vi "1-DSpecViewAndFit.vi"() -> ()   [LabVIEW 2022 SP3]
uses:
  <vilib>/Utility/file.llb/Read From Spreadsheet File (DBL).vi
  <vilib>/Utility/file.llb/Write To Spreadsheet File (DBL).vi
panel:
  in  "Extra File Att":dbl format="%.2f"
  out "single case fit data":T1 {"pts in fit" format="%.2f"; "midband fit" format="%.2f"; "intercept (b)" format="%.2f"; "slope (m)" format="%.3f"}
  in  "Log scaling?":bool=TRUE
  out "raw x coord":dbl[][](array[numeric]) format="%.2f"
  out "raw y coord":dbl[][](array[numeric]) format="%.2f"
  out "raw sector image":dbl[][](array[numeric]) format="%.2f"
  out "Axis scaling Params":T2 {"Y high" format="%.2f"; "Y low" format="%.2f"; "X left" format="%.2f"; "X right" format="%.2f"}
  out "Sector as data array":dbl[][](graph)
  in  "Last sector file":path
  in  "View Header?":bool
  in  "Save to Spectra.txt?":bool
  out "Cal File Att":string
  out "RF File Att":string
  in  "FFT size for":u16(ring)=6 items=["next 2^n", "8", "16", "32", "64", "128", "256", "512", "1024"]
  in  "Cal File Selection":u16(ring) items=["Don't subtract a Cal File", "Use Info in Header", "Specify Cal Info", "Make New Cal File"]
  in  "Cal File Name":string
  in  "Save New Cal File?":bool
  out "actual length\nof padded ROI":i32
  out "need this# of RF pts\nmatch Cal File":i32
  in  "Fit band":T3={"start"=3.5, "stop freq"=8.0, "center freq"=5.75} {"center freq" format="%.2f"; "stop freq" format="%.2f"; "start" format="%.2f"}
  out "Spectrum (dBr vs. MHz)":T4(graph)
  out "Raw data":i16[][](graph)
  in  "new eye file path":path
  # "Select region for spectrum analysis.\nKeep RED curser above and to left of blue.\nBath cursors can be on the same line."
  # "© 2000 Riverside Research Institute"
  # "Spectrum Fit Parameters"
  # "Blue curser controls upper right of sector ROI,\nRed curser controls lower left."
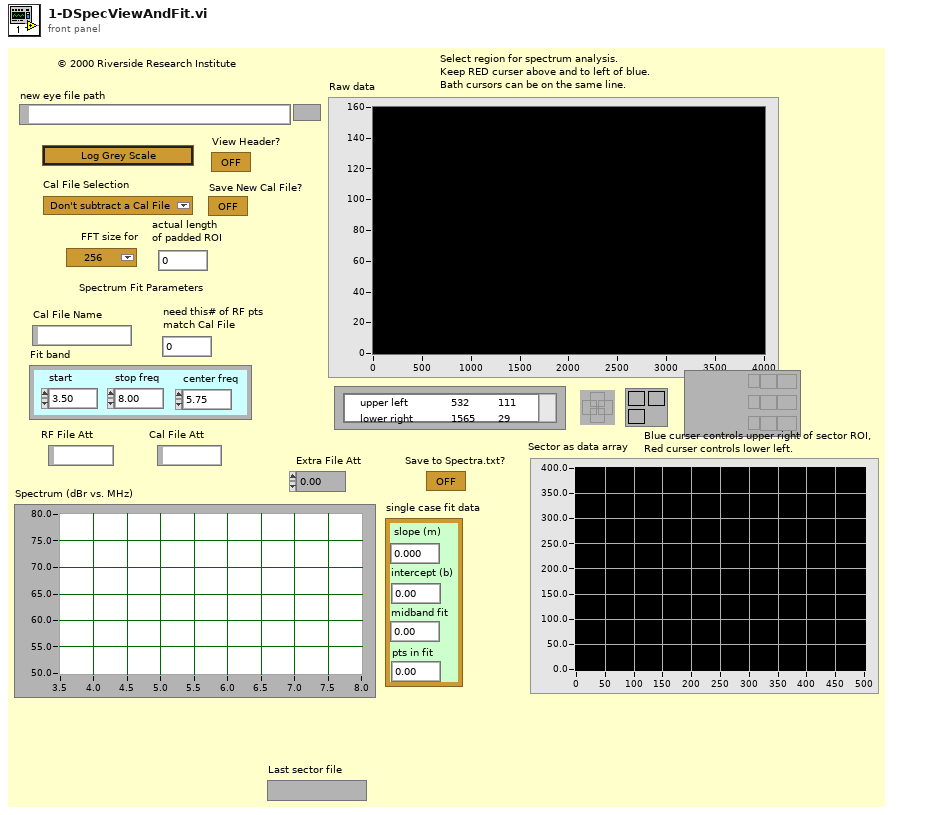
[diagram p1: front panel]
types:
  T1 = cluster{"slope (m)":dbl, "intercept (b)":dbl, "midband fit":dbl, "pts in fit":dbl}
  T2 = cluster{"X right":dbl, "X left":dbl, "Y low":dbl, "Y high":dbl}
  T3 = cluster{"start":dbl, "stop freq":dbl, "center freq":dbl}
  T4 = cluster{"fo of fit":dbl, "df (MHz)":dbl, "Best Linear Fit":dbl[]}[]
  T5 = cluster{"# rf points per line":u16, "# lines per scan":u16, "sample rate MHz":u16, "# A/D bits":u16, "# bytes per A/D":u16, "TGC Flag":u16, "A/D Type":string}
  T6 = cluster{"bandwidth":sgl, "center freq":sgl, "start freq":sgl, "ID":i32}
  T7 = cluster{"delay":sgl, "pivot distance":sgl, "sector scan angle":sgl, "operator":string, "Scan Mode":string, "location":string}
  T8 = cluster{"RF file name":string, "RF file att":string, "RF cal file name":string, "RF cal file att":string}
  T9 = cluster{"Cursor.Cursor X":dbl, dbl, "Cursor.Cursor Y":dbl, dbl}
  T10 = cluster{"Cursor.Cursor X":i32, i32, "Cursor.Cursor Y":i32, i32}
  T11 = cluster{"RF file name":string, "RF file att":string, "Cal File Name":string, "RF cal file att":string}
  T12 = cluster{"start freq":sgl, sgl, "center freq":sgl}
  T13 = cluster{"slope (m)":dbl[][], "intercept (b)":dbl[][], "midband fit":dbl[][], "pts in fit":dbl}
  T14 = cluster{"fo of fit":dbl, "df (MHz)":dbl, dbl[]}[]
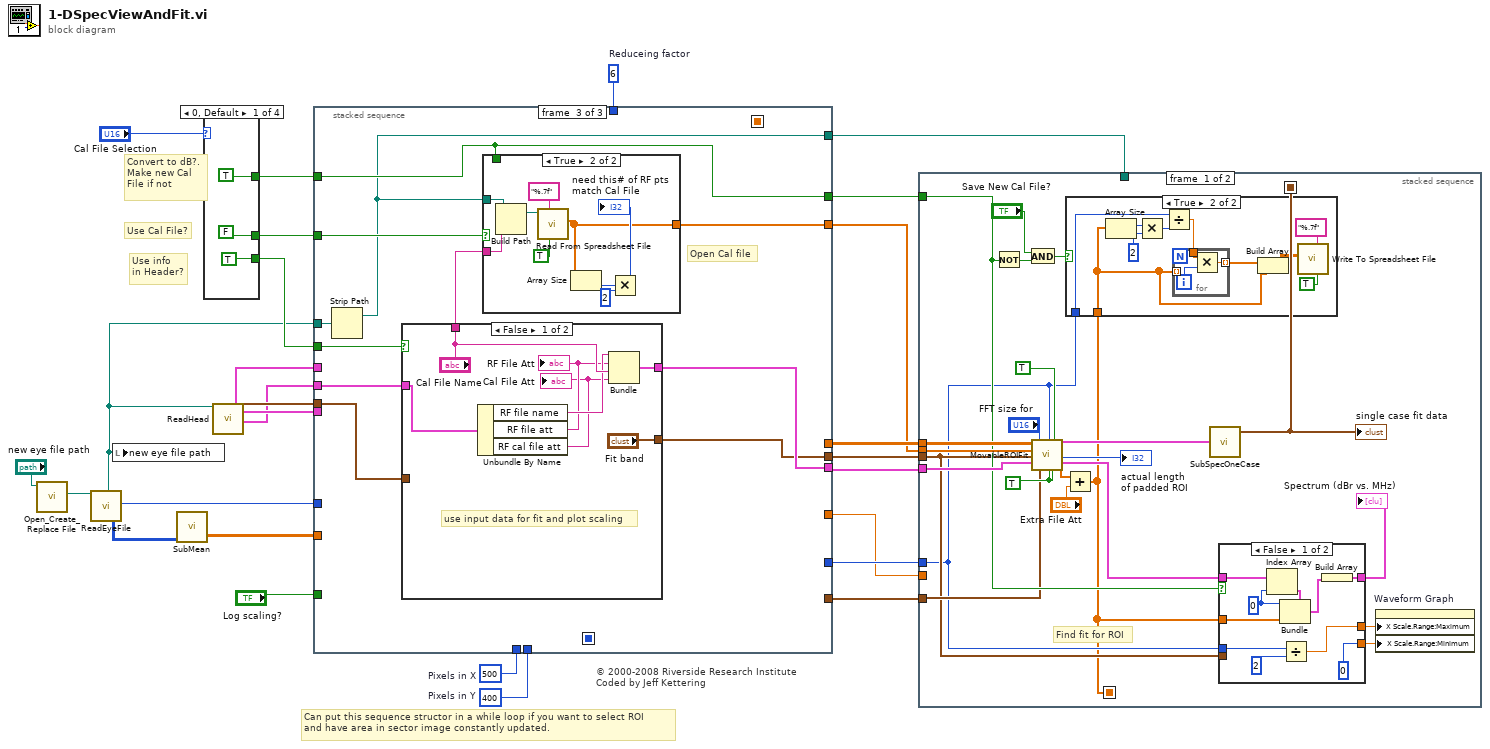
[diagram p0: block diagram]
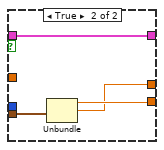
[diagram p2: hidden frame]
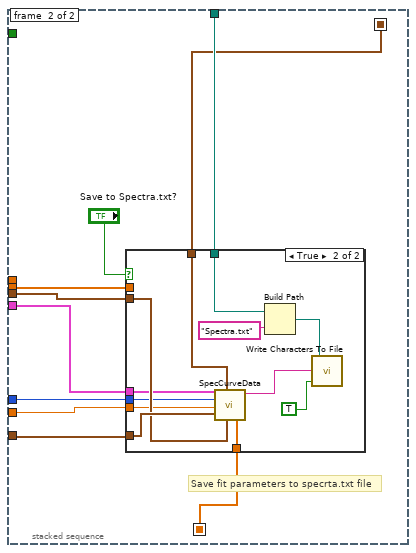
[diagram p4: hidden frame]
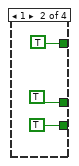
[diagram p6: hidden frame]
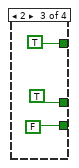
[diagram p7: hidden frame]
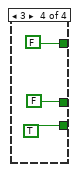
[diagram p8: hidden frame]
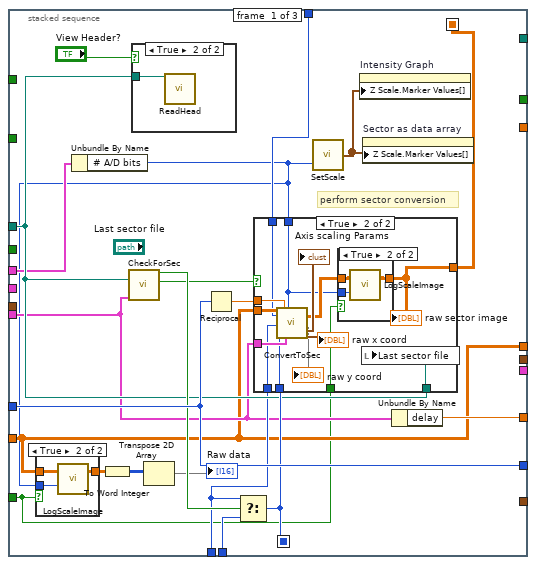
[diagram p9: hidden frame]
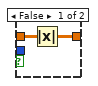
[diagram p10: hidden frame]
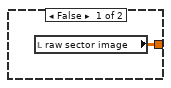
[diagram p12: hidden frame]
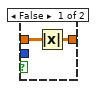
[diagram p13: hidden frame]
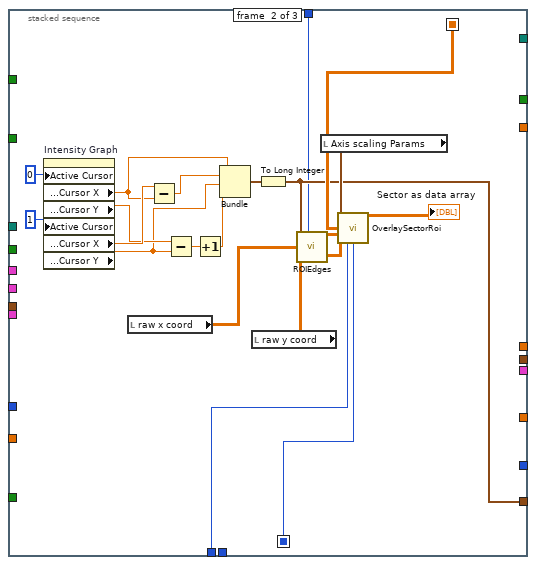
[diagram p14: hidden frame]
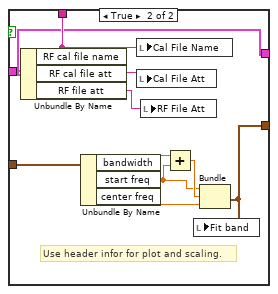
[diagram p15: hidden frame]
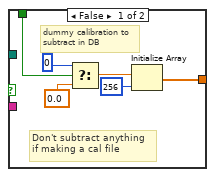
[diagram p16: hidden frame]
diagram:
  w7 = 400  # Pixels in Y
  w6 = 500  # Pixels in X
  w8 = 6  # Reduceing factor
  # "© 2000-2008 Riverside Research Institute\nCoded by Jeff Kettering"
  # "Can put this sequence structor in a while loop if you want to select ROI\nand have area in sector image constantly updated."
  # "Convert to dB?.\nMake new Cal\nFile if not"
  # "Use Cal File?"
  # "Use info\nin Header?"
  n1 = call <vilib>:"Open_Create_Replace File.vi"("file path"="new eye file path") -> ("new file path"=w13:path)  [unwired: 5 in, 5 out]
  n2 = call "ReadEyeFile.vi"("new file path"=w13) -> ("new path out"=w2:path, "2-D data array"=w3:i16[][], "sample rate MHz"=w23:u16)  [unwired: 1 in, 15 out]
  n3 = local write "new eye file path"(w2) -> ()
  n4 = call "SubMean.vi"("Scan Data In"=w3) -> ("Array"=w1:dbl[][])  [unwired: 3 in, 1 out]
  n5 = case shown="0, Default" "Cal File Selection" {
    tunnel: [TRUE TRUE TRUE FALSE] -> w26
    tunnel: [FALSE TRUE TRUE FALSE] -> w4
    tunnel: [TRUE TRUE FALSE TRUE] -> w25
    frame 0, Default {
    }
    frame 1 {
    }
    frame 2 {
    }
    frame 3 {
    }
  }
  n6 = call "ReadHead.vi"("new file path"=w2) -> ("A/D info"=w21:T5, "Tranducer Info"=w22:T6, "Scan Info"=w20:T7, "RF Info"=w19:T8)  [unwired: 15 out]
  n7 = stacked-sequence {
    seq-local: [w56 _ _] -> [_ w99 _]
    seq-local: [w53 _ _] -> [_ w97 _]
    tunnel: w26 -> [_ _ w111]
    tunnel: w4 -> [_ _ w117]
    tunnel: w25 -> [_ _ w116]
    tunnel: w23 -> [w59 _ _]
    tunnel: w1 -> [w45 _ _]
    tunnel: w22 -> [_ _ w115]
    tunnel: w21 -> [w48 _ _]
    tunnel: w20 -> [w47 _ _]
    tunnel: w19 -> [_ _ w114]
    tunnel: [_ _ w113] -> w15
    tunnel: [_ _ w110] -> w9
    tunnel: [_ w93 _] -> w16
    tunnel: [w57 _ _] -> w10
    tunnel: [w59 _ _] -> w12
    tunnel: [_ _ w109] -> w11
    tunnel: [_ _ w111] -> w18
    tunnel: [w45 _ _] -> w17
    tunnel: [_ _ w108] -> w14
    tunnel: w2 -> [w50 _ w112]
    tunnel: w8 -> [w55 w92 _]
    tunnel: w7 -> [w54 _ _]
    tunnel: w6 -> [w49 w94 _]
    tunnel: "Log scaling?" -> [w44 _ _]
    frame #0 {
      # "perform sector conversion"
      n8 = Unbundle By Name(w48) -> ("# A/D bits"=w43:u16)
      n9 = case shown="True" w44 {
        tunnel: w45 -> [w61 w65]
        tunnel: [w62 w64] -> w46
        tunnel: w43 -> [_ w63]
        frame False {
          n10 = Absolute Value(x=w61) -> (abs(x)=w62:dbl[][])
        }
        frame True {
          n11 = call "LogScaleImage.vi"("A/D bits"=w63, "input array"=w65) -> ("log scale image"=w64:dbl[][])  [unwired: 1 out]
        }
      }
      n12 = To Word Integer(number=w46) -> (16bit integer=w41:i16[][])
      n13 = call "CheckForSec.vi"("Scan Info"=w47, "Last sector file opened"=w50) -> ("sector?"=w51:bool, "= 360?"=w52:bool)  [unwired: 1 in, 5 out]
      n14 = case shown="True" "View Header?" {
        tunnel: w50 -> [_ w66]
        frame False {
        }
        frame True {
          n15 = call "ReadHead.vi"("new file path"=w66) -> ()  [unwired: 19 out]
        }
      }
      n16 = Transpose 2D Array(2D array=w41) -> (transposed array=→"Raw data":i16[][])
      n17 = Reciprocal(x=w59) -> (1/x=w60:dbl)
      n18 = Select(t=w49, s=w52, f=w54) -> (s? t:f=w53:i32)
      n19 = case shown="True" w51 {
        tunnel: [w67 w70] -> w56
        tunnel: w45 -> [_ w81]
        tunnel: w47 -> [_ w80]
        tunnel: w60 -> [_ w79]
        tunnel: w50 -> [_ w78]
        tunnel: w55 -> [_ w74]
        tunnel: w49 -> [_ w73]
        tunnel: w53 -> [_ w72]
        tunnel: w44 -> [_ w69]
        tunnel: w43 -> [_ w68]
        frame False {
          n20 = local read "raw sector image"() -> (w67:dbl[][])
        }
        frame True {
          n21 = call "ConvertToSec.vi"("raw image data in"=w81, "reduce pts by factor of"=w74, "pixels in x"=w73, "pixels in y"=w72, "Time between rf pts\nmicros"=w79, "Scan Info"=w80, "Abs?"=w68) -> (13:→"raw y coord", "raw sector out"=w71:dbl[][], "Axis scaling Params"=→"Axis scaling Params":T2, "scales"=→"raw x coord":cluster{"inc x (mm)":dbl, "inc y (mm)":dbl})  [unwired: 4 in, 5 out]
          n22 = case shown="True" w69 {
            tunnel: w71 -> [w83 w86]
            tunnel: [w82 w85] -> w70
            tunnel: w68 -> [_ w84]
            frame False {
              n23 = Absolute Value(x=w83) -> (abs(x)=w82:dbl[][])
            }
            frame True {
              n24 = call "LogScaleImage.vi"("A/D bits"=w84, "input array"=w86) -> ("log scale image"=w85:dbl[][])  [unwired: 1 out]
            }
          }
          "raw sector image" <- w70
          n25 = local write "Last sector file"(w78) -> ()
        }
      }
      n26 = call "SetScale.vi"("# A/D bits"=w43) -> ("Array"=w42:cluster{dbl, u32}[])  [unwired: 1 in]
      n27 = property on="Intensity Graph" class="IntGraph (strict)"("Z Scale.Marker Values[]"=w42) -> ()  [unwired: 2 in, 2 out]
      n28 = property on="Sector as data array" class="IntGraph (strict)"("Z Scale.Marker Values[]"=w42) -> ()  [unwired: 2 in, 2 out]
      n29 = Unbundle By Name(w47) -> ("delay"=w57:sgl)
    }
    frame #1 {
      n30 = property on="Intensity Graph" class="IntGraph (strict)"("Active Cursor"=u32 0 ("Write Attribute"), "Active Cursor"=u32 1 ("Write Attribute")) -> ("Cursor.Cursor Position:Cursor X"=w103:dbl, "Cursor.Cursor Position:Cursor Y"=w106:dbl, "Cursor.Cursor Position:Cursor X"=w107:dbl, "Cursor.Cursor Position:Cursor Y"=w102:dbl)  [unwired: 2 in, 2 out]
      n31 = local read "raw x coord"() -> (w91:dbl[][])
      n32 = Subtract(x=w107, y=w103) -> (x-y=w87:dbl)
      n33 = Subtract(x=w106, y=w102) -> (x-y=w101:dbl)
      n34 = Increment(x=w101) -> (x+1=w88:dbl)
      n35 = Bundle("Cursor.Cursor X"=w103, w87, "Cursor.Cursor Y"=w102, w88) -> (w100:T9)  [unwired: 1 out]
      n36 = local read "raw y coord"() -> (w98:dbl[][])
      n37 = To Long Integer(number=w100) -> (32bit integer=w93:T10)
      n38 = call "ROIEdges.vi"("Array Subset"=w93, "reduce pts by factor of"=w92, "raw x coord"=w91, "raw y coord"=w98) -> ("x box"=w90:dbl[][], "y box"=w89:dbl[][])  [unwired: 1 in]
      n39 = local read "Axis scaling Params"() -> (w96:T2)
      n40 = call "OverlaySectorRoi.vi"("Axis scaling Params"=w96, "Sector as Array"=w99, "x coord"=w90, "y coord"=w89, "pixels in x"=w94, "pixels in y"=w97) -> ("image overlay"=→"Sector as data array":dbl[][])  [unwired: 2 in, 7 out]
    }
    frame #2 {
      # "Open Cal file"
      n41 = Strip Path(path=w112) -> (stripped path=w110:path)  [unwired: 1 out]
      n42 = case shown="False" w116 {
        tunnel: w115 -> [_ w135]
        tunnel: ["Fit band" w132] -> w108
        tunnel: w114 -> [w122 w128]
        tunnel: ["Cal File Name" w129] -> w118
        tunnel: [w124 w128] -> w109
        frame False {
          # "use input data for fit and plot scaling"
          n43 = Unbundle By Name(w122) -> ("RF file name"=w121:string, "RF file att"=w120:string, "RF cal file att"=w119:string)
          "RF File Att" <- w120
          "Cal File Att" <- w119
          n44 = Bundle("RF file name"=w121, "RF file att"=w120, "Cal File Name"="Cal File Name", "RF cal file att"=w119) -> (w124:T11)  [unwired: 1 out]
        }
        frame True {
          # "Use header infor for plot and scaling."
          n45 = Unbundle By Name(w128) -> ("RF cal file name"=w129:string, "RF cal file att"=w127:string, "RF file att"=w126:string)
          n46 = Unbundle By Name(w135) -> ("bandwidth"=w134:sgl, "start freq"=w130:sgl, "center freq"=w133:sgl)
          n47 = local write "Cal File Name"(w129) -> ()
          n48 = local write "Cal File Att"(w127) -> ()
          n49 = local write "RF File Att"(w126) -> ()
          n50 = Add(x=w134, y=w130) -> (x+y=w131:sgl)
          n51 = Bundle("start freq"=w130, w131, "center freq"=w133) -> (w132:T12)  [unwired: 1 out]
          n52 = local write "Fit band"(w132) -> ()
        }
      }
      n53 = case shown="True" w117 {
        tunnel: w118 -> [_ w150]
        tunnel: w111 -> [w139 _]
        tunnel: w110 -> [_ w143]
        tunnel: [w136 w142] -> w113
        frame False {
          # "Don't subtract anything\nif making a cal file"
          # "dummy calibration to\nsubtract in DB"
          n54 = Select(t=0, s=w139, f=0.0 ("t")) -> (s? t:f=w138:dbl)
          n55 = Initialize Array(w138, 256 ("Dimension Size")) -> (w136:dbl[])
        }
        frame True {
          n56 = Build Path(base path=w143, name or relative path=w150) -> (appended path=w149:path)
          n57 = call-poly <vilib>:"Read From Spreadsheet File.vi"("transpose (no:F)"=TRUE, "format (%.3f)"="%.7f", "file path (dialog if empty)"=w149) -> ("first row"=w142:dbl[])  [unwired: 1 in, 7 out]
          n58 = Array Size(array=w142) -> (size(s)=w147:i32)
          n59 = Multiply(x=w147, y=2) -> (x*y=→"need this# of RF pts\nmatch Cal File":i32)
        }
      }
    }
  }
  n60 = stacked-sequence {
    seq-local: [w162 _] -> [_ w202]
    seq-local: [w151 _] -> [_ w201]
    tunnel: w18 -> [w159 _]
    tunnel: w17 -> [w170 _]
    tunnel: w16 -> [w158 w209]
    tunnel: w15 -> [w166 w210]
    tunnel: w14 -> [w157 w208]
    tunnel: w12 -> [w154 w207]
    tunnel: w11 -> [w163 w206]
    tunnel: w10 -> [_ w205]
    tunnel: w9 -> [_ w203]
    frame #0 {
      w173 = TRUE
      # "Find fit for ROI"
      n61 = Not(x=w159) -> (.not. x?=w168:bool)
      n62 = And(x="Save New Cal File?", y=w168) -> (x .and. y?=w167:bool)
      n63 = call "MovableROIFit.vi"("input array"=w170, "calibration data"=w166, "Fit band"=w157, "RF Info"=w163, "FFT size for"="FFT size for", "Fit array"=w158, "freq (MHz)"=w154, "Single ROI?"=w173, "subtract spectrum\nfrom fit?"=TRUE ("subtract spectrum\nfrom fit?"), "convert output to dB?"=w173) -> ("Raw Fit Data"=w165:T13, "Length of padded array"=→"actual length\nof padded ROI":i32, "Plots"=w161:T14, "power spectrum in dB"=w153:dbl[])  [unwired: 3 in, 3 out]
      n64 = Add(x=w153, y="Extra File Att") -> (x+y=w151:dbl[])
      n65 = case shown="True" w167 {
        tunnel: w151 -> [_ w188]
        tunnel: w154 -> [_ w195]
        frame False {
        }
        frame True {
          n66 = Array Size(array=w188) -> (size(s)=w194:i32)
          n67 = Multiply(x=w194, y=2) -> (x*y=w193:i32)
          n68 = Divide(x=w195, y=w193) -> (x/y=w191:dbl)
          n69 = for {
            tunnel: w188 -> [_] mode=indexing
            tunnel: w191 -> [w199]
            tunnel: [w198] -> w190 mode=indexing
            i -> [w200]
            n70 = Multiply(x=w199, y=w200) -> (x*y=w198:dbl)
          }
          n71 = Build Array(w190, w188) -> (w189:dbl[][])
          n72 = call-poly <vilib>:"Write To Spreadsheet File.vi"("transpose? (no:F)"=TRUE, "format (%.3f)"="%.7f", "2D data"=w189) -> ()  [unwired: 3 in, 3 out]
        }
      }
      n73 = call "SubSpecOneCase.vi"("Raw Fit Data"=w165) -> ("single case fit data"=w162:T1)  [unwired: 3 in, 5 out]
      "single case fit data" <- w162
      n74 = case shown="False" w159 {
        tunnel: w161 -> [w183 w187]
        tunnel: [w181 w187] -> w160
        tunnel: w151 -> [w182 _]
        tunnel: w157 -> [_ w186]
        tunnel: [w177 w184] -> w156
        tunnel: [0 w185] -> w155
        tunnel: w154 -> [w178 _]
        frame False {
          w180 = 0
          n75 = Index Array(array=w183, index=w180) -> (element=w174:cluster{"fo of fit":dbl, "df (MHz)":dbl, dbl[]})
          n76 = Bundle(cluster=w174, "fo of fit"=w180, w182) -> (w175:cluster{"fo of fit":dbl, "df (MHz)":dbl, dbl[]})  [unwired: 1 out]
          n77 = Divide(x=w178, y=2) -> (x/y=w177:dbl)
          n78 = Build Array(w175) -> (w181:T14)
        }
        frame True {
          n79 = Unbundle(w186) -> ("start"=w185:dbl, "stop freq"=w184:dbl)  [unwired: 1 out]
        }
      }
      "Spectrum (dBr vs. MHz)" <- w160
      n80 = property on="Waveform Graph" class="WFGraph (strict)"("X Scale.Range:Maximum"=w156, "X Scale.Range:Minimum"=w155) -> ()  [unwired: 2 in, 2 out]
    }
    frame #1 {
      # "Save fit parameters to specrta.txt file"
      n81 = case shown="True" "Save to Spectra.txt?" {
        tunnel: w210 -> [_ _]
        tunnel: w209 -> [_ w218]
        tunnel: w208 -> [_ w217]
        tunnel: w207 -> [_ w216]
        tunnel: w206 -> [_ w215]
        tunnel: w205 -> [_ w214]
        tunnel: w203 -> [_ w213]
        tunnel: w202 -> [_ w212]
        tunnel: w201 -> [_ w211]
        frame False {
        }
        frame True {
          n82 = call "SpecCurveData.vi"("spectal data"=w211, "Fit band"=w217, "Fit params"=w212, "Array Subset"=w218, "delay"=w214, "sample rate MHz"=w216, "RF Info"=w215) -> ("Spectra data"=w219:string)  [unwired: 4 out]
          n83 = Build Path(base path=w213, name or relative path="Spectra.txt") -> (appended path=w221:path)
          n84 = call <vilib>:"Write Characters To File.vi"("append to file? (new file:F)"=TRUE, "character string"=w219, "file path (dialog if empty)"=w221) -> ()  [unwired: 3 out]
        }
      }
    }
  }
